vi "Close Account.vi"(8 "entrée d'erreur":errorcluster, 11 "Infos sur le compte":T1) -> (0 "sortie d'erreur":errorcluster)   [LabVIEW 2013]
uses:
  Account Info.ctl
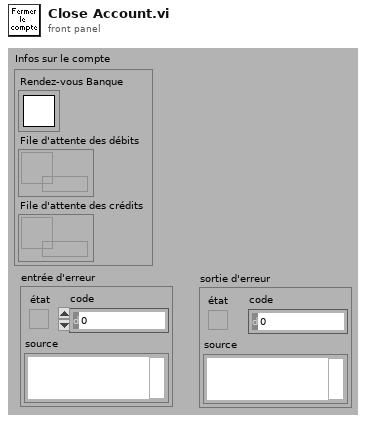
[diagram p1: front panel]
types:
  T1 = typedef "Account Info.ctl" = cluster{"Rendez-vous Banque":T2, "File d'attente des débits":refnum<queue>, "File d'attente des crédits":refnum<queue>}
  T2 = typedef "Rendezvous RefNum" = refnum<k1>
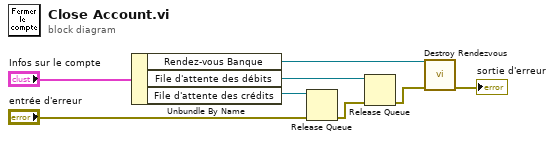
[diagram p0: block diagram]
diagram:
  n1 = Unbundle By Name ("Désassembler par nom")("Infos sur le compte") -> ("Rendez-vous Banque"=w7:T2, "File d'attente des débits"=w4:refnum<queue>, "File d'attente des crédits"=w6:refnum<queue>)
  n2 = Release Queue ("Libérer une file d'attente")(queue=w6, error in (no error)="entrée d'erreur") -> (error out=w5:errorcluster)  [unwired: 3 out]
  n3 = Release Queue ("Libérer une file d'attente")(queue=w4, error in (no error)=w5) -> (error out=w3:errorcluster)  [unwired: 3 out]
  n4 = call <vilib>:"Destroy Rendezvous.vi"("error in (no error)"=w3, "rendezvous"=w7) -> ("error out"=→"sortie d'erreur":errorcluster)  [unwired: 5 out]
